vi "getWavelength_v80AM8.vi"() -> ()   [LabVIEW 2016]
uses:
  <vilib>/Analysis/baseanly.llb/Mean (DBL).vi
  FPGA/Stats/Stats/StatsLV/WavemeterPauseGlobal.vi
  <vilib>/Analysis/NI_AALBase.lvlib
  x32/CLDevIFace.dll
panel:
  out "Wavelength":dbl format="%0.5f"
  out "0.75ppm in Wave (nm)":dbl format="%#_3g"
  out "0.75ppm in Freq (MHz)":dbl
  out "Freq (Hz)":dbl
  out "standard dev":dbl format="%0.5f"
  in  "# for Stdev":i32=7
  in  "Avg":i32=1
  out "Delta MHz":dbl
  in  "Scale Factor":dbl=800.0
  out "Power (mW)":dbl format="%.9f"
  in  "Clear Chart?":bool
  in  "Delay Time (s)":dbl=0.01
  out "Wavelength vs time":cluster{dbl[], dbl[]}(graph)
  out "error out":errorcluster
  out "output param":i32
  in  "stop":bool
  in  "OK Button":bool
  in  "CommPort":dbl=5.0 caption="Comm Port #"
  # "Pr = 605.977"
  # "Super cavity FSR  6 GHz\nZerodure FSR  750 MHz"
  # "1 pm = 200 MHz @1212nm\n1 pm = 800 MHz @606 nm"
  # "Bristol 621B accuracy = 0.75 ppm\nuseful conversions:"
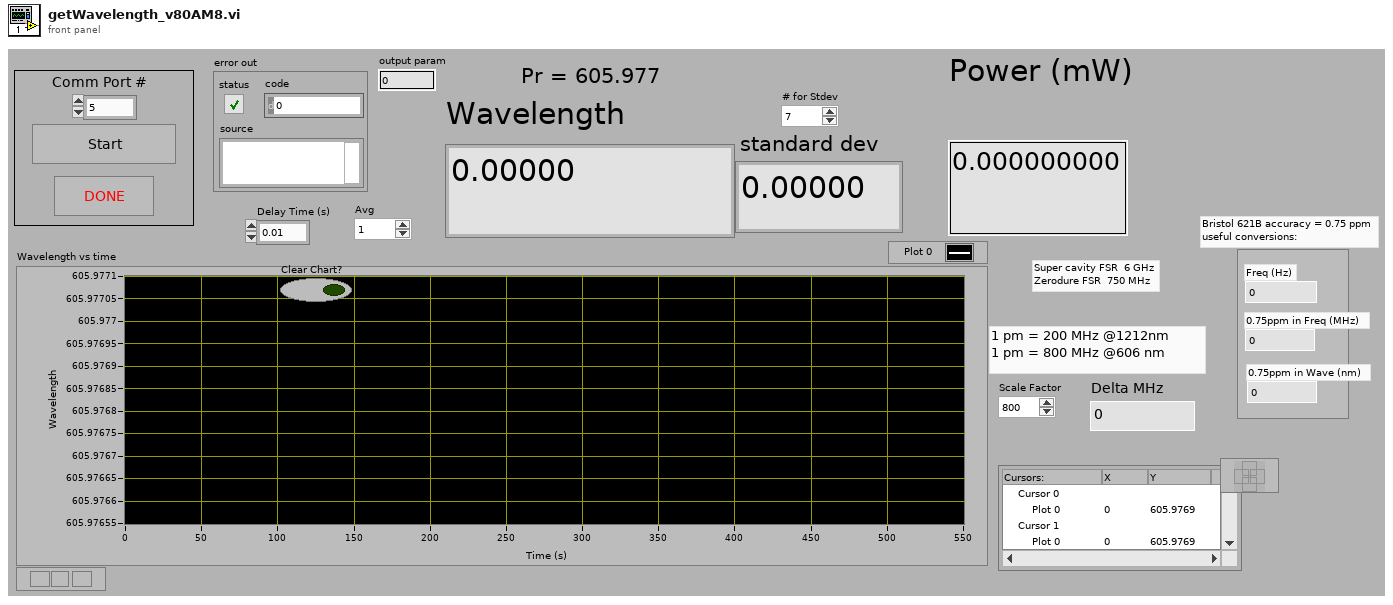
[diagram p1: front panel]
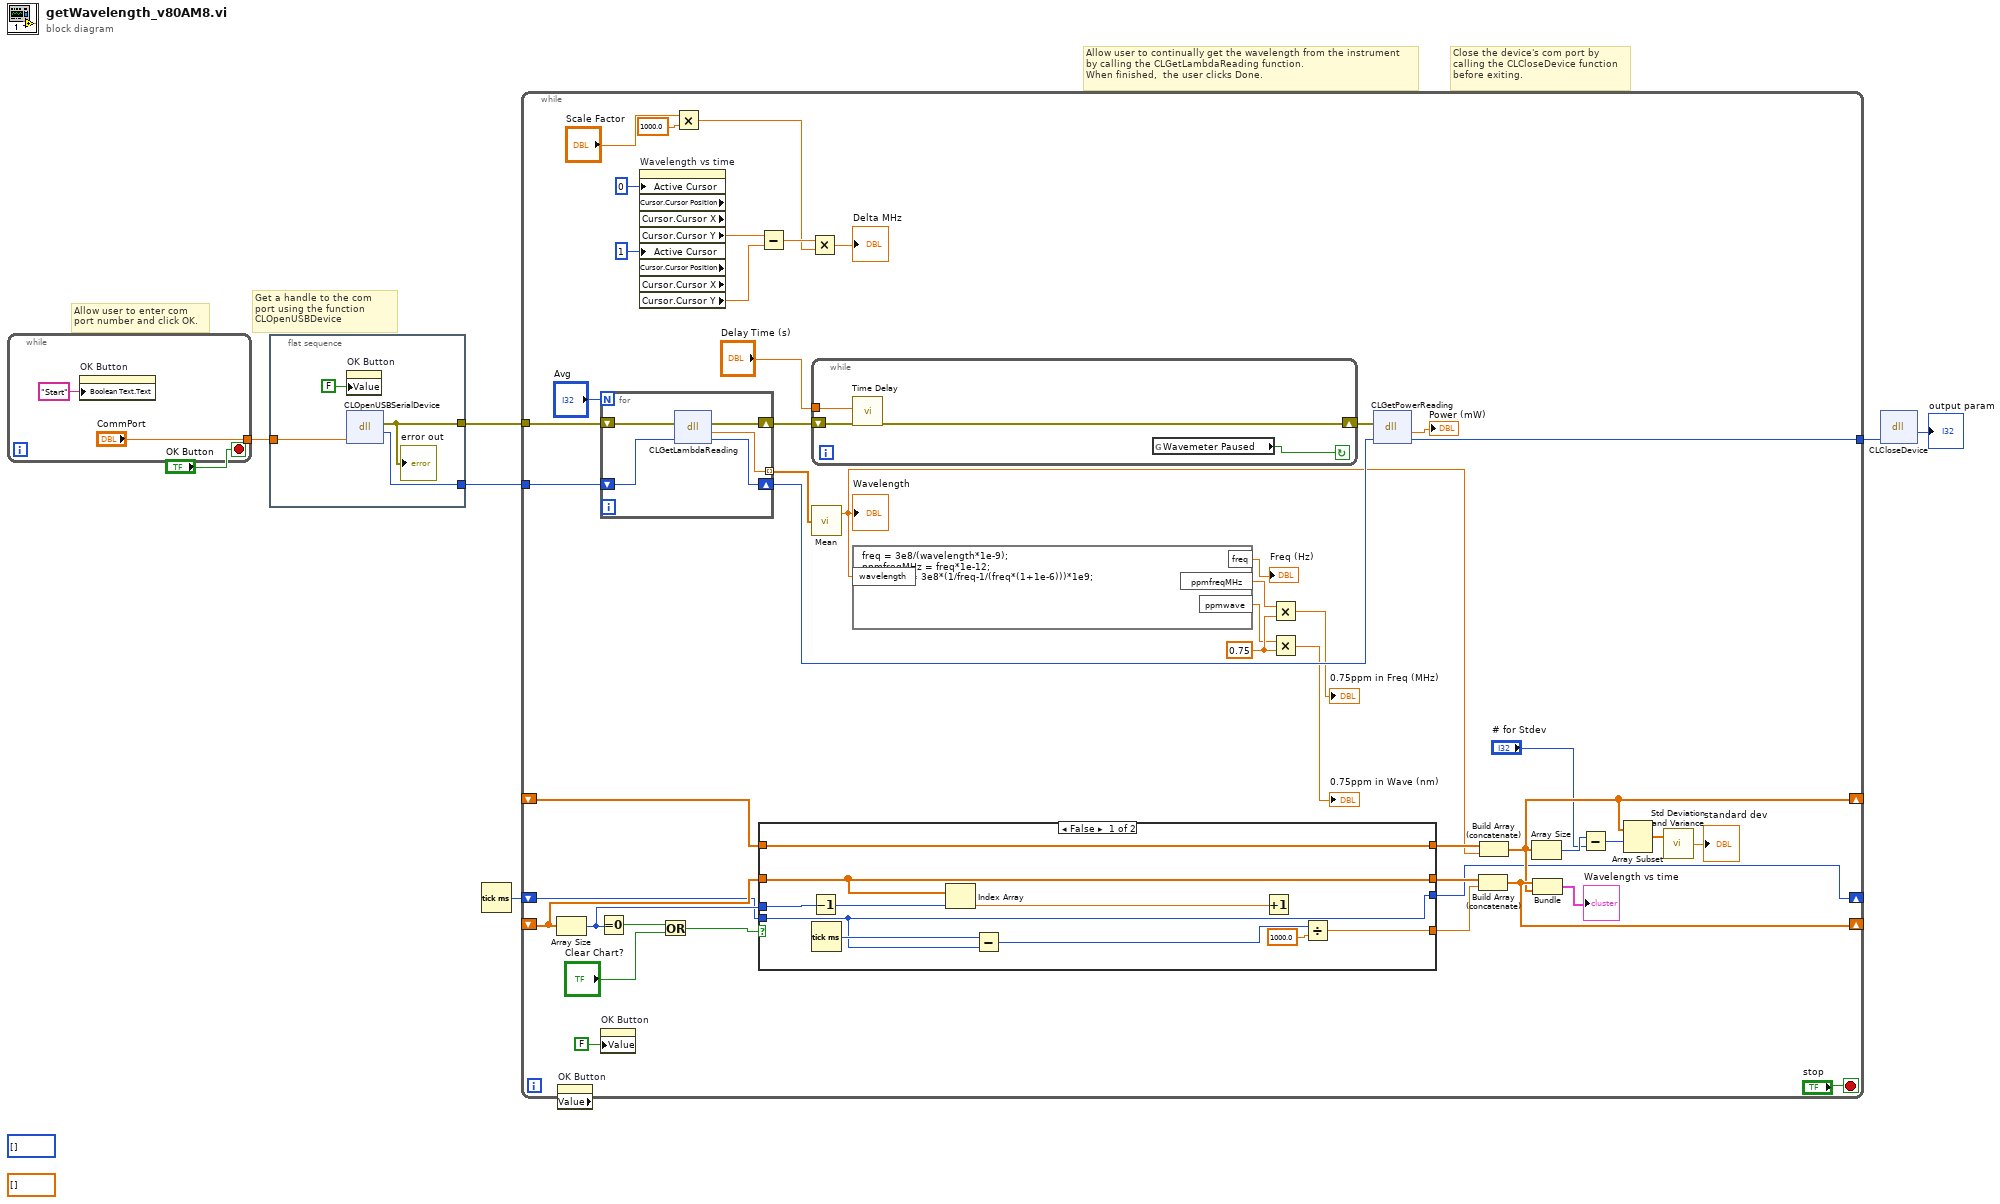
[diagram p0: block diagram]
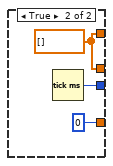
[diagram p2: hidden frame]
diagram:
  (unwired) i32[] []
  (unwired) dbl[] []
  # "Close the device's com port by\ncalling the CLCloseDevice function\nbefore exiting."
  # "Allow user to continually get the wavelength from the instrument\nby calling the CLGetLambdaReading function.  \nWhen finished,  the user clicks Done."
  # "Get a handle to the com\nport using the function CLOpenUSBDevice"
  # "Allow user to enter com \nport number and click OK."
  n1 = while {
    tunnel: ["CommPort"] -> w6
    stop <- "OK Button" stop-if-true
    n2 = property on="OK Button" class="Bool (strict)"("Boolean Text.Text"="Start") -> ()  [unwired: 2 in, 2 out]
  }
  n3 = flat-sequence {
    tunnel: w6 -> [w13]
    tunnel: [w12] -> w5
    tunnel: [w10] -> w2
    frame #0 {
      n4 = property on="OK Button" class="Bool (strict)"("Value"=FALSE) -> ()  [unwired: 2 in, 2 out]
      n5 = dll-call lib="C:/Users/Lab/Desktop/Bristol wavemeter 621/00424-2-00 621 customer CD/Programming Interface/x32/CLDevIFace.dll" fn="CLOpenUSBSerialDevice"("commPort"=w13) -> (error out=w10:errorcluster, "return type"=w12:i32)  [unwired: 4 in, 1 out]
      "error out" <- w10
    }
  }
  n6 = Tick Count (ms)() -> (millisecond timer value=w1:u32)
  n7 = while {
    tunnel: w5 -> [w60]
    tunnel: [w48] -> w4
    shift-right: [w28] -> _
    shift-left: _ -> [w52]
    shift-right: [w57] -> _
    shift-left: _ -> [w33]
    tunnel: w2 -> [w53]
    shift-right: [w14] -> _
    shift-left: w1 -> [w15]
    stop <- "stop" stop-if-true
    w18 = 0.75 ("y")
    n8 = Array Size(array=w33) -> (size(s)=w30:i32)
    n9 = property on="OK Button" class="Bool (strict)" props=["Value"]() -> ()  [unwired: 2 in, 3 out]
    n10 = Equal To 0?(x=w30) -> (x = 0?=w38:bool)
    n11 = for {
      N: "Avg" -> [_]
      tunnel: [w68] -> w31 mode=indexing
      shift-right: [w65] -> w49
      shift-left: w60 -> [w69]
      shift-right: [w67] -> w54
      shift-left: w53 -> [w66]
      n12 = dll-call lib="C:/Users/Lab/Desktop/Bristol wavemeter 621/00424-2-00 621 customer CD/Programming Interface/x32/CLDevIFace.dll" fn="CLGetLambdaReading"(error in=w66, "devHandle"=w69) -> (error out=w67:errorcluster, "return type"=w68:dbl, "devHandle"=w65:i32)  [unwired: 2 in, 1 out]
    }
    n13 = property on="OK Button" class="Bool (strict)"("Value"=FALSE) -> ()  [unwired: 2 in, 2 out]
    n14 = property on="Wavelength vs time" class="XYGraph (strict)" props=["Active Cursor", "Cursor", "Cursor Position", "Cursor", "Cursor X", "Cursor", "Cursor Y", "Active Cursor", "Cursor", "Cursor Position", "Cursor", "Cursor X", "Cursor", "Cursor Y"]("Active Cursor"=u32 0, "Active Cursor"=u32 1) -> ("Cursor.Cursor Y"=w44:dbl, "Cursor.Cursor Y"=w45:dbl)  [unwired: 2 in, 6 out]
    n15 = Or(x=w38, y="Clear Chart?") -> (x .or. y?=w36:bool)
    n16 = Multiply(x="Scale Factor", y=1000.0) -> (x*y=w39:dbl)
    n17 = Subtract(x=w44, y=w45) -> (x-y=w46:dbl)
    n18 = case shown="False" w36 {
      tunnel: w52 -> [w79 _]
      tunnel: w33 -> [w78 _]
      tunnel: [w78 w80] -> w34
      tunnel: [w79 w80] -> w35
      tunnel: w30 -> [w76 _]
      tunnel: [w71 0] -> w29
      tunnel: w15 -> [w70 _]
      tunnel: [w70 w81] -> w14
      frame False {
        n19 = Decrement(x=w76) -> (x-1=w75:i32)
        n20 = Tick Count (ms)() -> (millisecond timer value=w74:u32)
        n21 = Index Array(array=w78, index=w75) -> (element=w77:dbl)
        n22 = Subtract(x=w74, y=w70) -> (x-y=w72:u32)
        n23 = Increment(x=w77) -> ()  [unwired: 1 out]
        n24 = Divide(x=w72, y=1000.0) -> (x/y=w71:dbl)
      }
      frame True {
        w80 = dbl[] []
        n25 = Tick Count (ms)() -> (millisecond timer value=w81:u32)
      }
    }
    n26 = Multiply(x=w46, y=w39) -> (x*y=→"Delta MHz":dbl)
    n27 = while {
      tunnel: "Delay Time (s)" -> [w64]
      shift-right: [w62] -> w51
      shift-left: w54 -> [w63]
      stop <- w61 continue-if-true
      n28 = call "Time Delay"("error in (no error)"=w63, "Delay Time (s)"=w64) -> ("error out"=w62:errorcluster)  [unwired: 9 in]
      n29 = global read "WavemeterPauseGlobal.vi" "Wavemeter Paused"() -> (w61:bool)
    }
    n30 = call-poly <vilib>:"Mean.vi"("X"=w31) -> ("mean"=w21:dbl)  [unwired: 1 out]
    "Wavelength" <- w21
    n31 = formula code="freq = 3e8/(wavelength*1e-9);\nppmfreqMHz = freq*1e-12;\nppmwave = 3e8*(1/freq-1/(freq*(1+1e-6)))*1e9;"("wavelength"=w21) -> ("freq"=→"Freq (Hz)":dbl, "ppmfreqMHz"=w20:dbl, "ppmwave"=w17:dbl)
    n32 = Multiply(x=w20, y=w18) -> (x*y=→"0.75ppm in Freq (MHz)":dbl)
    n33 = Multiply(x=w17, y=w18) -> (x*y=→"0.75ppm in Wave (nm)":dbl)
    n34 = dll-call lib="C:/Users/Lab/Desktop/Bristol wavemeter 621/00424-2-00 621 customer CD/Programming Interface/x32/CLDevIFace.dll" fn="CLGetPowerReading"(error in=w51, "devHandle"=w49) -> ("return type"=→"Power (mW)":dbl, "devHandle"=w48:i32)  [unwired: 2 in, 2 out]
    n35 = Build Array (concatenate)(w34, w29) -> (w57:dbl[])
    n36 = Build Array (concatenate)(w35, w21) -> (w28:dbl[])
    n37 = Array Size(array=w28) -> (size(s)=w27:i32)
    n38 = Bundle(w57, w28) -> (→"Wavelength vs time":cluster{dbl[], dbl[]})  [unwired: 1 in]
    n39 = Subtract(x=w27, y="# for Stdev") -> (x-y=w25:i32)
    n40 = Array Subset(array=w28, index=w25) -> (w24:dbl[])  [unwired: 1 in]
    n41 = call <vilib>:"Std Deviation and Variance.vi"("X"=w24) -> ("standard deviation"=→"standard dev":dbl)  [unwired: 1 in, 2 out]
  }
  n42 = dll-call lib="C:/Users/Lab/Desktop/Bristol wavemeter 621/00424-2-00 621 customer CD/Programming Interface/x32/CLDevIFace.dll" fn="CLCloseDevice"("commPort"=w4) -> ("return type"=→"output param":i32)  [unwired: 4 in, 2 out]
